vi "StatusSetRegister.vi"(7 "Val":i32 format="%.0g", 8 "error in (no error)":errorcluster {"code" format="%.0x"}, 9 "SubRegister (Condition)":i32(ring) items=["Condition", "Negative Transition", "Positive Transition", "Event", "Enable"], 10 "Register (Status Byte)":i32(ring) items=["Status Byte"=0, "Standard Event"=1, "Operation"=2, "Questionable"=3, "Status Register Operation Condition"=4, "Status Register Operation Enable"=5, "Status Register Operation Event"=6, "Status Register Operation Instrument Condition"=16, "Status Register Operation Instrument Enable"=17, "Status Register Operation Instrument Event"=18, "Status Register Operation Instrument Negative Transition"=19, "Status Register Operation Instrument Positive Transition"=20, "Status Register Operation Negative Transition"=7, "Status Register Operation Positive Transition"=8, "Status Register Questionable Calibration Condition"=21, "Status Register Questionable Calibration Enable"=22, "Status Register Questionable Calibration Event"=23, "Status Register Questionable Calibration Extended Failure Condition"=24, "Status Register Questionable Calibration Extended Failure Enable"=25, "Status Register Questionable Calibration Extended Failure Event"=26, "Status Register Questionable Calibration Extended Failure Negative Transition"=27, "Status Register Questionable Calibration Extended Failure Positive Transition"=28, "Status Register Questionable Calibration Extended Needed Condition"=29, "Status Register Questionable Calibration Extended Needed Enable"=30, "Status Register Questionable Calibration Extended Needed Event"=31, "Status Register Questionable Calibration Extended Needed Negative Transition"=32, "Status Register Questionable Calibration Extended Needed Positive Transition"=33, "Status Register Questionable Calibration Negative Transition"=34, "Status Register Questionable Calibration Positive Transition"=35, "Status Register Questionable Calibration Skipped Condition"=36, "Status Register Questionable Calibration Skipped Enable"=37, "Status Register Questionable Calibration Skipped Event"=38, "Status Register Questionable Calibration Skipped Negative Transition"=39, "Status Register Questionable Calibration Skipped Positive Transition"=40, "Status Register Questionable Condition"=9, "Status Register Questionable Enable"=10, "Status Register Questionable Event"=11, "Status Register Questionable Frequency Condition"=41, "Status Register Questionable Frequency Enable"=42, "Status Register Questionable Frequency Event"=43, "Status Register Questionable Frequency Negative Transition"=44, "Status Register Questionable Frequency Positive Transition"=45, "Status Register Questionable Integrity Condition"=46, "Status Register Questionable Integrity Enable"=47, "Status Register Questionable Integrity Event"=48, "Status Register Questionable Integrity Negative Transition"=49, "Status Register Questionable Integrity Positive Transition"=50, "Status Register Questionable Integrity Signal Condition"=51, "Status Register Questionable Integrity Signal Enable"=52, "Status Register Questionable Integrity Signal Event"=53, "Status Register Questionable Integrity Signal Negative Transition"=54, "Status Register Questionable Integrity Signal Positive Transition"=55, "Status Register Questionable Integrity Un Calibrated Condition"=56, "Status Register Questionable Integrity Un Calibrated Enable"=57, "Status Register Questionable Integrity Un Calibrated Event"=58, "Status Register Questionable Integrity Un Calibrated Negative Transition"=59, "Status Register Questionable Integrity Un Calibrated Positive Transition"=60, "Status Register Questionable Negative Transition"=12, "Status Register Questionable Positive Transition"=13, "Status Register Questionable Power Condition"=61, "Status Register Questionable Power Enable"=62, "Status Register Questionable Power Event"=63, "Status Register Questionable Power Negative Transition"=64, "Status Register Questionable Power Positive Transition"=65, "Status Register Questionable Temperature Condition"=66, "Status Register Questionable Temperature Enable"=67, "Status Register Questionable Temperature Event"=68, "Status Register Questionable Temperature Negative Transition"=69, "Status Register Questionable Temperature Positive Transition"=70, "Status Register Service Request Enable"=14, "Status Register Standard Event Enable"=15], 11 "instrument handle":refnum<k15>) -> (0 "error out":errorcluster, 3 "instrument handle out":refnum<k15>)   [LabVIEW 2009, in "Keysight XSAn.lvlib"]
doc: "Insturment status registers.\n\nSupported Models: All supported"
uses:
  <instrlib>/Keysight XSAn/Keysight XSAn.lvlib
  AgXSAn.dll
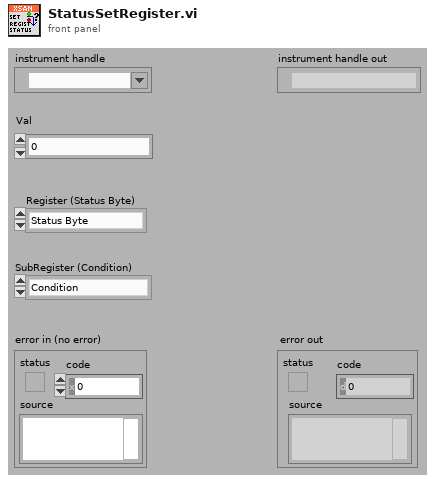
[diagram p1: front panel]
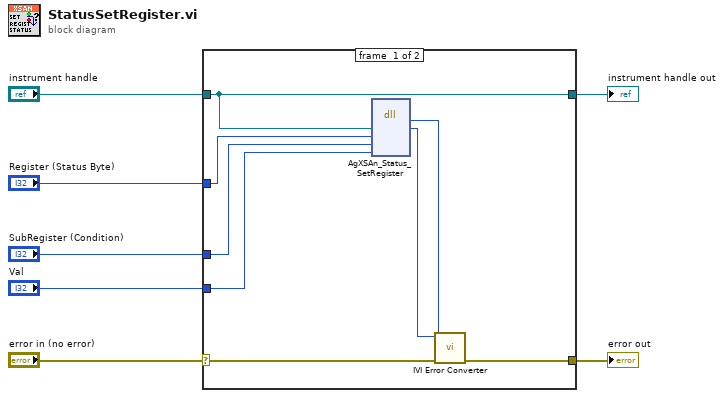
[diagram p0: block diagram]
diagram:
  n1 = case shown="No Error" "error in (no error)" {
    selector: "error in (no error)" -> [w13 w17]
    tunnel: [w12 w17] -> w7
    tunnel: "instrument handle" -> [w9 w16]
    tunnel: "SubRegister (Condition)" -> [w11 _]
    tunnel: "Val" -> [w10 _]
    tunnel: [w9 w16] -> w2
    tunnel: "Register (Status Byte)" -> [w8 _]
    frame #0 {
      n2 = dll-call lib="AgXSAn**.dll" fn="AgXSAn_Status_SetRegister"("Vi"=w9, "Register"=w8, "SubRegister"=w11, "Val"=w10) -> (w14:i32, "Vi"=w15:u32)  [unwired: 6 in, 2 out]
      n3 = call <instrlib>:"IVI Error Converter.vi"("error in (no error)"=w13, "IVI error code (0)"=w14, "instrument handle"=w15) -> ("error out"=w12:errorcluster)  [unwired: 7 in, 1 out]
    }
    frame #1 {
    }
  }
  "error out" <- w7
  "instrument handle out" <- w2
